vi "startup include.vi"(6 "LabVIEW Web Service":refnum<class "Web Service.lvclass">) -> ()   [LabVIEW 2013]
uses:
  <vilib>/wsapi/Web Service.lvclass
  execution/Tag Bus Web Interface runtime.lvclass
  configuration/Tag Bus Web Interface configuration.lvclass
  execution/close.vi
  execution/output.vi
  execution/classify error.vi
  execution/input.vi
  execution/init.vi
  configuration/validate.vi
  configuration/to string.vi
  configuration/subtable.ctl
  configuration/from string.vi
  configuration/set channel.vi
  configuration/rename channel.vi
  configuration/get channels.vi
  configuration/delete channel from configuration.vi
  configuration/apply channel changes.vi
  configuration/add channel to configuration.vi
  configuration/data table to subtable.vi
  configuration/get supported types.vi
  configuration/Get Supported Targets.vi
  configuration/instance count allowed.vi
  configuration/execution class name.vi
  configuration/Write channels.vi
  configuration/Read channels.vi
panel:
  # "Use the web service input terminal to call the VIs on the Service subpalette of the Web Services palette. Do not remove it from the connector pane unless you don't need access to the palette."
  # "Any additional terminals added to the connector pane of a startup VI will be ignored."
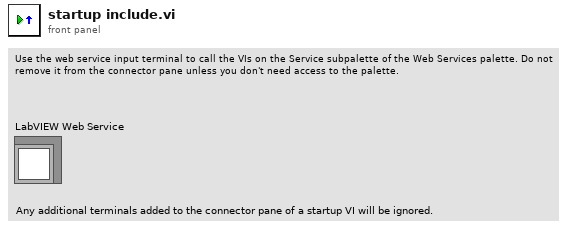
[diagram p1: front panel]
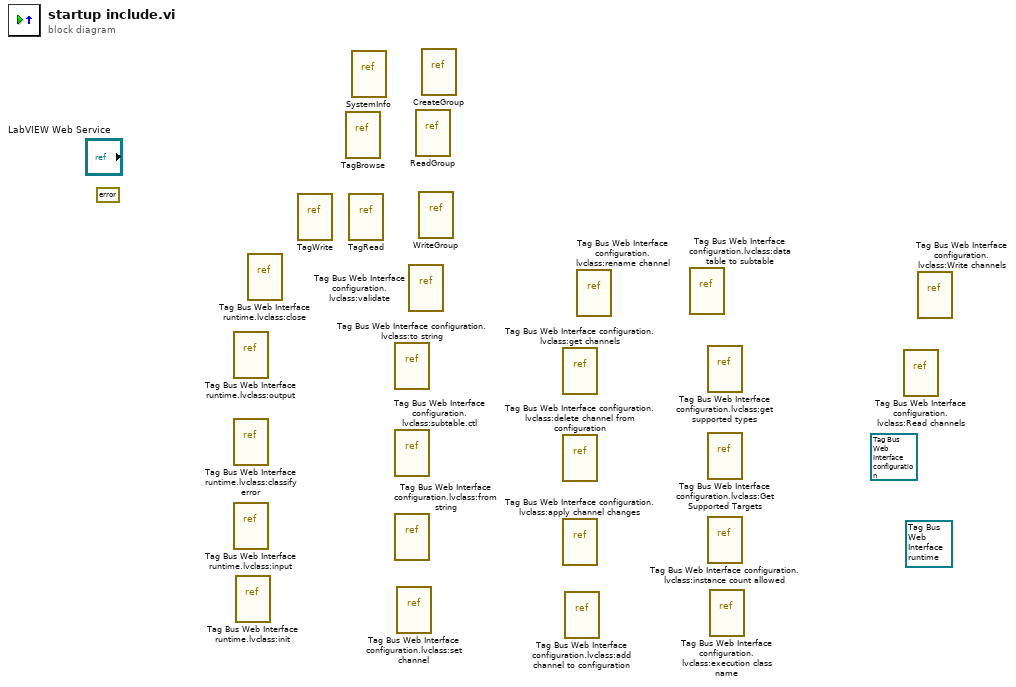
[diagram p0: block diagram]
diagram:
  (unwired) refnum<class "Tag Bus Web Interface configuration.lvclass"> refnum ("Tag Bus Web Interface configuration")
  (unwired) refnum<class "Tag Bus Web Interface runtime.lvclass"> refnum ("Tag Bus Web Interface runtime")
  (unwired) errorcluster {"status"=FALSE, "code"=0, "source"=""} ("error constant")
  n1 = vi-ref "Tag Bus Web Interface runtime.lvclass:output.vi"() -> ()  [unwired: 1 out]
  n2 = vi-ref "Tag Bus Web Interface runtime.lvclass:classify error.vi"() -> ()  [unwired: 1 out]
  n3 = vi-ref "Tag Bus Web Interface runtime.lvclass:input.vi"() -> ()  [unwired: 1 out]
  n4 = vi-ref "Tag Bus Web Interface runtime.lvclass:init.vi"() -> ()  [unwired: 1 out]
  n5 = vi-ref "Tag Bus Web Interface runtime.lvclass:close.vi"() -> ()  [unwired: 1 out]
  n6 = vi-ref "TagWrite.vi"() -> ()  [unwired: 1 out]
  n7 = vi-ref "TagBrowse.vi"() -> ()  [unwired: 1 out]
  n8 = vi-ref "TagRead.vi"() -> ()  [unwired: 1 out]
  n9 = vi-ref "SystemInfo.vi"() -> ()  [unwired: 1 out]
  n10 = vi-ref "Tag Bus Web Interface configuration.lvclass:to string.vi"() -> ()  [unwired: 1 out]
  n11 = vi-ref "Tag Bus Web Interface configuration.lvclass:subtable.ctl"() -> ()  [unwired: 1 out]
  n12 = vi-ref "Tag Bus Web Interface configuration.lvclass:from string.vi"() -> ()  [unwired: 1 out]
  n13 = vi-ref "Tag Bus Web Interface configuration.lvclass:set channel.vi"() -> ()  [unwired: 1 out]
  n14 = vi-ref "Tag Bus Web Interface configuration.lvclass:validate.vi"() -> ()  [unwired: 1 out]
  n15 = vi-ref "ReadGroup.vi"() -> ()  [unwired: 1 out]
  n16 = vi-ref "WriteGroup.vi"() -> ()  [unwired: 1 out]
  n17 = vi-ref "CreateGroup.vi"() -> ()  [unwired: 1 out]
  n18 = vi-ref "Tag Bus Web Interface configuration.lvclass:get channels.vi"() -> ()  [unwired: 1 out]
  n19 = vi-ref "Tag Bus Web Interface configuration.lvclass:delete channel from configuration.vi"() -> ()  [unwired: 1 out]
  n20 = vi-ref "Tag Bus Web Interface configuration.lvclass:apply channel changes.vi"() -> ()  [unwired: 1 out]
  n21 = vi-ref "Tag Bus Web Interface configuration.lvclass:add channel to configuration.vi"() -> ()  [unwired: 1 out]
  n22 = vi-ref "Tag Bus Web Interface configuration.lvclass:rename channel.vi"() -> ()  [unwired: 1 out]
  n23 = vi-ref "Tag Bus Web Interface configuration.lvclass:data table to subtable.vi"() -> ()  [unwired: 1 out]
  n24 = vi-ref "Tag Bus Web Interface configuration.lvclass:get supported types.vi"() -> ()  [unwired: 1 out]
  n25 = vi-ref "Tag Bus Web Interface configuration.lvclass:Get Supported Targets.vi"() -> ()  [unwired: 1 out]
  n26 = vi-ref "Tag Bus Web Interface configuration.lvclass:instance count allowed.vi"() -> ()  [unwired: 1 out]
  n27 = vi-ref "Tag Bus Web Interface configuration.lvclass:execution class name.vi"() -> ()  [unwired: 1 out]
  n28 = vi-ref "Tag Bus Web Interface configuration.lvclass:Read channels.vi"() -> ()  [unwired: 1 out]
  n29 = vi-ref "Tag Bus Web Interface configuration.lvclass:Write channels.vi"() -> ()  [unwired: 1 out]
